vi "CAN Transceiver Test.vi"() -> ()   [LabVIEW 2024]
uses:
  Shared Modules/CAN Commands Interpreter/XNET Session Settings.ctl
  Shared Modules/CAN Commands Interpreter/CAN Frame Data.ctl
  Shared Modules/CAN Commands Interpreter/Command Values.ctl
  Type Definitions/Tester States.ctl
  Shared Modules/CAN Commands Interpreter/Target Sessions - Initialize Output Session.vi
  Shared Modules/CAN Commands Interpreter/Target Sessions - Initialize Input Session.vi
  Shared Modules/CAN Commands Interpreter/Target Sessions - Start Session.vi
  Shared Modules/CAN Commands Interpreter/Target Sessions - Stop Session.vi
  Shared Modules/CAN Commands Interpreter/Target Sessions - Clear Session.vi
  Shared Modules/CAN Commands Interpreter/CAN Commands.lvlib
panel:
  in  "Tab Control":enum32{"Sessions", "Monitor", "Errors"}(tab)
  in  "Tester Sessions":T1[](array[typedef])=[{"Interface"="CAN2", "Frame List"=["ECU_Responses\nCAN Dataframes", "HeartBit\nCAN Dataframes", "Crank_Angle\nCAN Dataframes", "Throttle\nCAN Dataframes"], "Session ID"="", "Session Name"="Tester - Read ECU Responses"}, {"Interface"="CAN2", "Frame List"=["Tester_Requests\nCAN Dataframes"], "Session ID"="", "Session Name"="Tester - Write Requests"}, {"Interface"="CAN2", "Frame List"=["HeartBit\nCAN Dataframes"], "Session ID"="", "Session Name"="Tester - Write Heartbit"}]
  out "Read ECU Data":T2[][](array[typedef]) {"ID" format="%01x"; "Payload" format="%02x"}
  in  "Command":T3={"Command"="Enable Voltage Out", "Value"=0.0}
  in  "Send Command to ECU":bool
  out "Working Mode":T4=enum."Init"
  out "Reading?":bool
  in  "STOP":bool
  out "ECU Found":bool
  out "ECU Connected":bool
  in  "Connect":bool
  in  "Disconnect":bool
  in  "Restart":bool
  out "Write Error":errorcluster
  out "Read Error":errorcluster
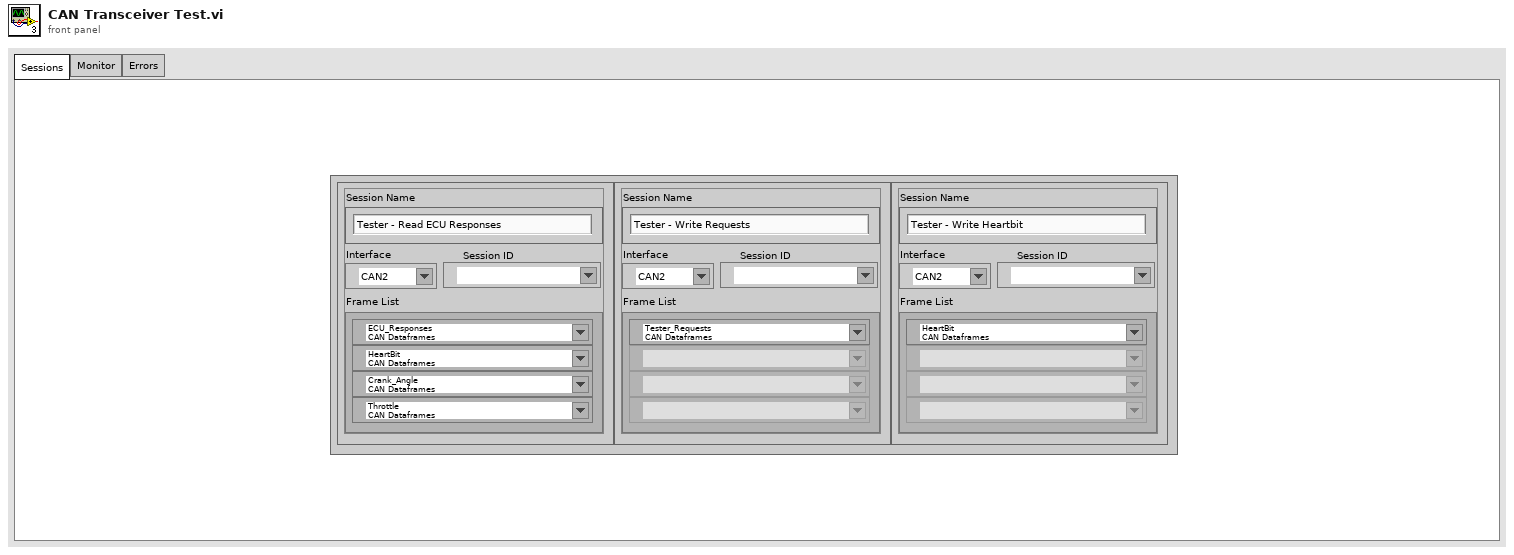
[diagram p1: front panel]
types:
  T1 = typedef "CAN Commands.lvlib/XNET Session Settings.ctl" = cluster{"Interface":refnum<k21>, "Frame List":refnum<k21>[], "Session ID":refnum<k21>, "Session Name":string}
  T2 = typedef "CAN Commands.lvlib/CAN Frame Data.ctl" = cluster{"Command":string, "XNET Frame":refnum<k21>, "Payload":u8[], "ID":u32, "Time Stamp":timestamp}
  T3 = typedef "CAN Commands.lvlib/Command Values.ctl" = cluster{"Command":string, "Value":dbl}
  T4 = typedef "Tester States.ctl" = enum16{"IDLE", "Init", "Monitoring", "Testing", "Wait for Reconnect", "Restart", "End"}
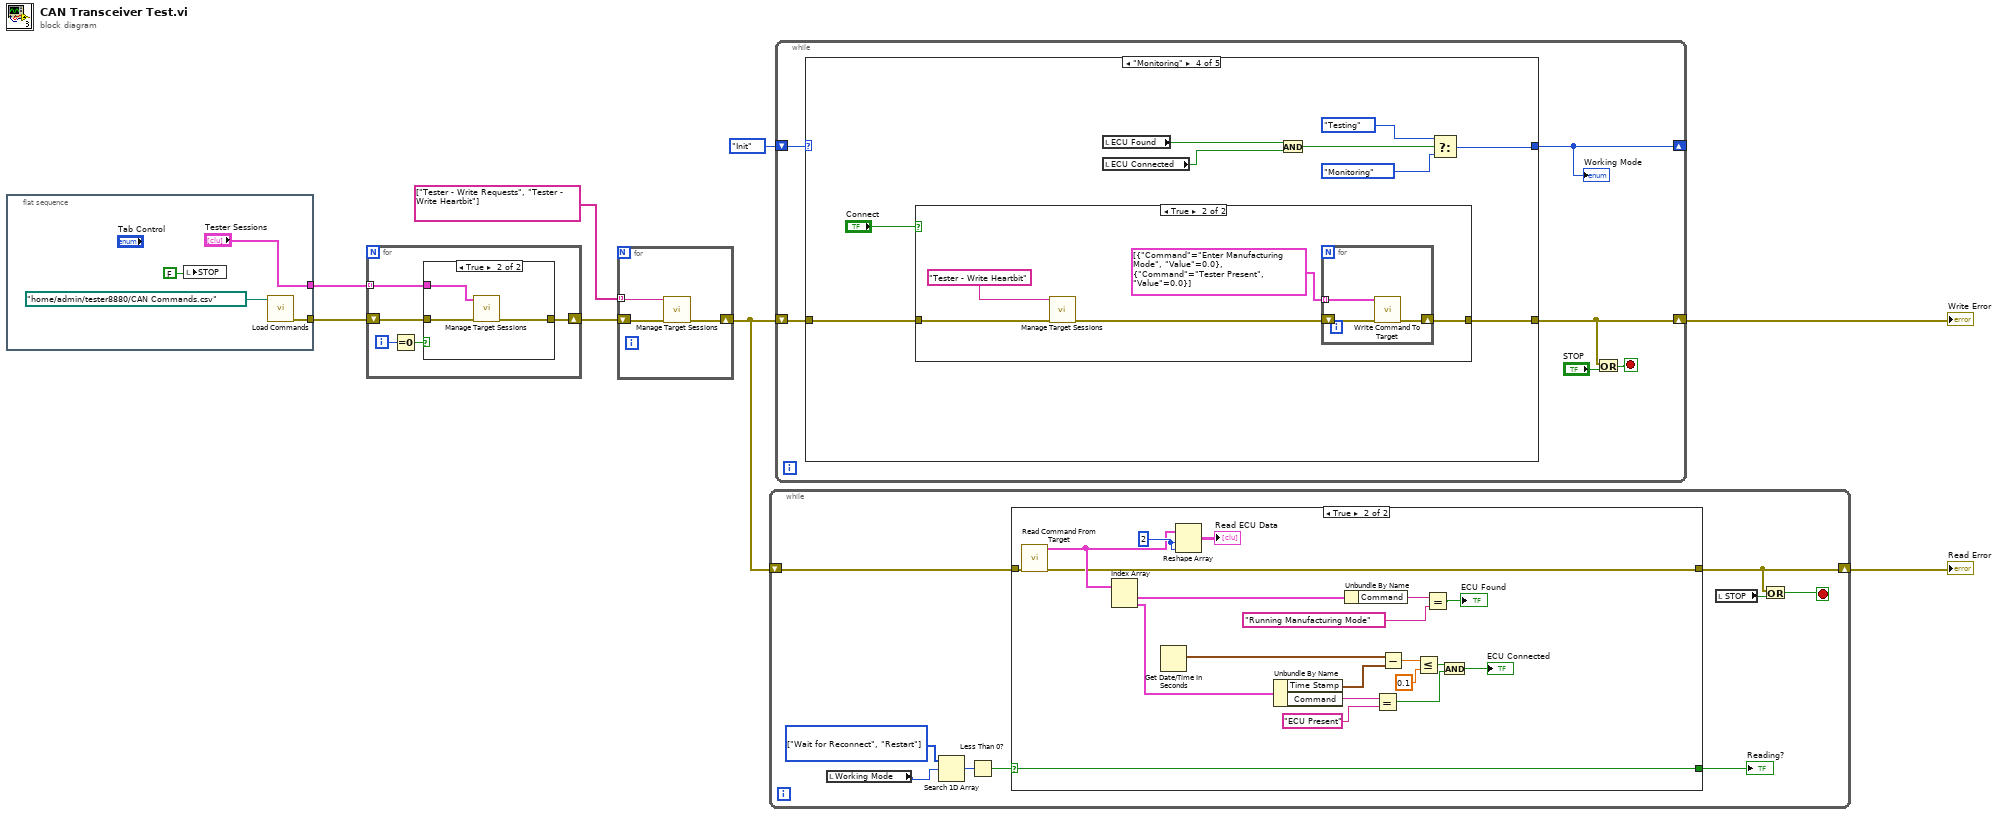
[diagram p0: block diagram]
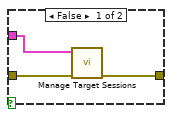
[diagram p2: hidden frame]
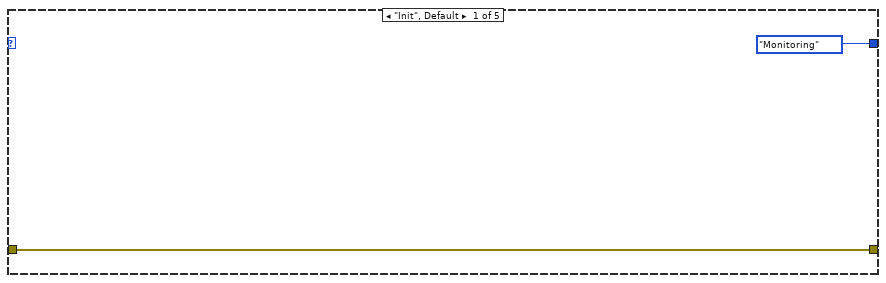
[diagram p3: hidden frame]
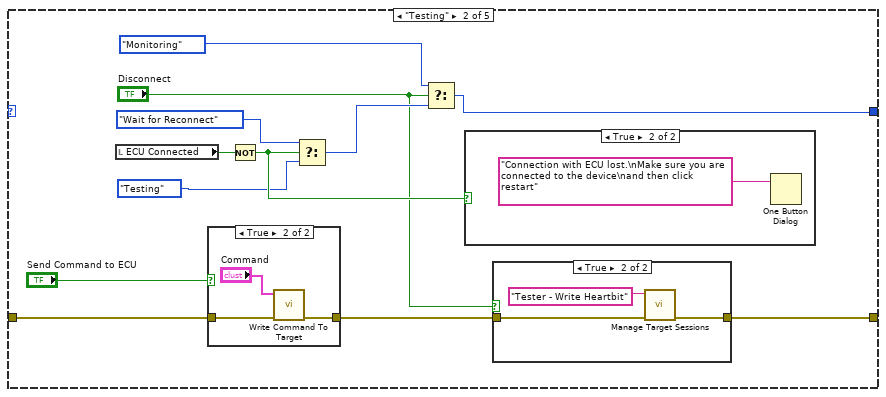
[diagram p4: hidden frame]
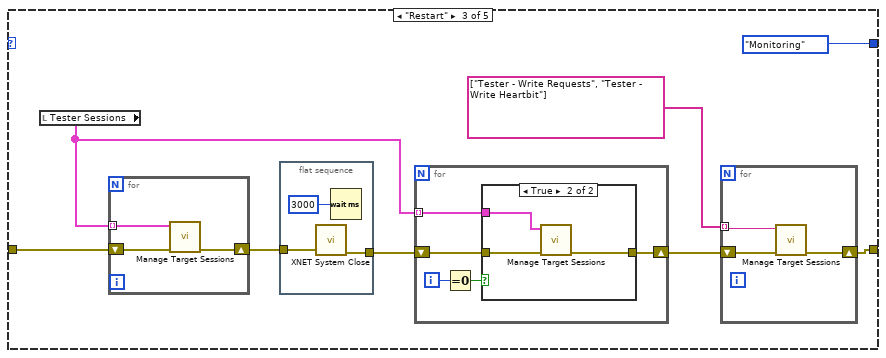
[diagram p8: hidden frame]
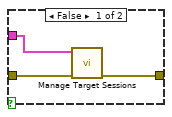
[diagram p9: hidden frame]
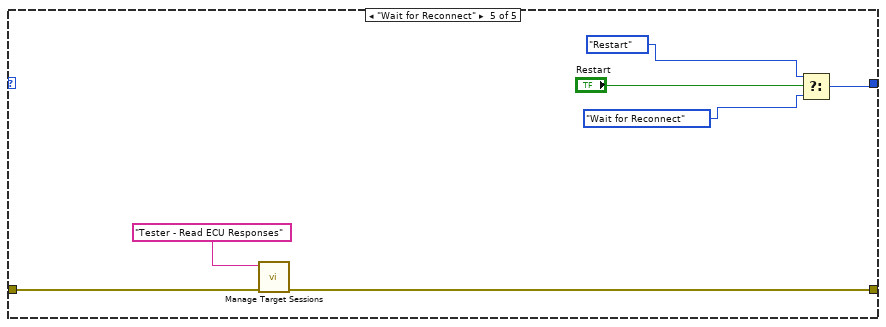
[diagram p11: hidden frame]
diagram:
  n1 = flat-sequence {
    tunnel: [w11] -> w8
    tunnel: ["Tester Sessions"] -> w4
    frame #0 {
      n2 = local write "STOP"(FALSE ("STOP")) -> ()
      n3 = call "Load Commands.vi"("Commands File (CSV)"=path "/home/admin/tester8880/CAN Commands.csv") -> ("error out"=w11:errorcluster)  [unwired: 10 in]
    }
  }
  n4 = for {
    shift-right: [w17] -> w7
    shift-left: w8 -> [w16]
    tunnel: w4 -> [w15] mode=indexing
    i -> [w13]
    n5 = Equal To 0?(x=w13) -> (x = 0?=w14:bool)
    n6 = case shown="True" w14 {
      tunnel: [w19 w23] -> w17
      tunnel: w16 -> [w20 w22]
      tunnel: w15 -> [w18 w21]
      frame False {
        n7 = call-poly "Manage Target Sessions.vi"("error in"=w20, "XNET Session Resouces"=w18) -> ("error out"=w19:errorcluster)  [unwired: 9 in]
      }
      frame True {
        n8 = call-poly "Manage Target Sessions.vi"("error in"=w22, "XNET Session Resouces"=w21) -> ("error out"=w23:errorcluster)  [unwired: 9 in]
      }
    }
  }
  n9 = for {
    shift-right: [w26] -> w1
    shift-left: w7 -> [w25]
    tunnel: string[] ["Tester - Write Requests", "Tester - Write Heartbit"] -> [w24] mode=indexing
    n10 = call-poly "Manage Target Sessions.vi"("error in"=w25, "Session Name"=w24) -> ("error out"=w26:errorcluster)  [unwired: 9 in]
  }
  n11 = while {
    shift-right: [w33] -> w5
    shift-left: w1 -> [w35]
    stop <- w32 stop-if-true
    w30 = T4[] [enum."Wait for Reconnect", enum."Restart"] items=["IDLE", "Init", "Monitoring", "Testing", "Wait for Reconnect", "Restart", "End"]
    n12 = local read "Working Mode"() -> (w29:T4)
    n13 = Search 1D Array(1D array=w30, element=w29) -> (index of element=w28:i32)  [unwired: 1 in]
    n14 = Less Than 0?(x=w28) -> (x < 0?=w27:bool)
    n15 = case shown="True" w27 {
      selector: w27 -> [_ w37]
      tunnel: w35 -> [w36 w56]
      tunnel: [w36 w38] -> w33
      tunnel: [_ w37] -> w31
      frame False {
      }
      frame True {
        w55 = 2 ("dimension size")
        n16 = call "Read Command From Target.vi"("error in"=w56) -> ("error out"=w38:errorcluster, "XNET Data"=w41:T2[])  [unwired: 7 in, 2 out]
        n17 = Index Array(array=w41) -> (element #1=w53:T2, element #2=w42:T2)  [unwired: 2 in]
        n18 = Get Date/Time In Seconds() -> (seconds since 1Jan1904=w40:timestamp)
        n19 = Reshape Array(w41, w55, w55) -> (→"Read ECU Data":T2[][])
        n20 = Unbundle By Name(w42) -> ("Time Stamp"=w43:timestamp, "Command"=w47:string)
        n21 = Unbundle By Name(w53) -> ("Command"=w52:string)
        n22 = Equal?(x=w47, y="ECU Present") -> (x = y?=w49:bool)
        n23 = Subtract(x=w40, y=w43) -> (x-y=w44:dbl)
        n24 = Less Or Equal?(x=w44, y=0.1) -> (x <= y?=w46:bool)
        n25 = Equal?(x=w52, y="Running Manufacturing Mode") -> (x = y?=→"ECU Found":bool)
        n26 = And(x=w46, y=w49) -> (x .and. y?=→"ECU Connected":bool)
      }
    }
    "Reading?" <- w31
    n27 = local read "STOP"() -> (w34:bool)
    n28 = Or(x=w33, y=w34) -> (x .or. y?=w32:bool)
  }
  "Read Error" <- w5
  n29 = while {
    shift-right: [w57] -> _
    shift-left: Tester_States."Init" -> [w62]
    shift-right: [w59] -> w2
    shift-left: w1 -> [w61]
    stop <- w58 stop-if-true
    n30 = case shown="\"Monitoring\"" w62 {
      tunnel: [Tester_States."Monitoring" w73 Tester_States."Monitoring" w118 w138] -> w57
      tunnel: [w64 w69 w87 w121 w135] -> w59
      tunnel: w61 -> [w64 w76 w88 w122 w136]
      frame "Init", Default {
      }
      frame "Testing" {
        n31 = local read "ECU Connected"() -> (w72:bool)
        n32 = case shown="True" "Send Command to ECU" {
          tunnel: w76 -> [w82 w85]
          tunnel: [w82 w84] -> w68
          frame False {
          }
          frame True {
            n33 = call "Write Command To Target.vi"("error out"=w85, "Command"="Command") -> ("error out"=w84:errorcluster)  [unwired: 9 in]
          }
        }
        n34 = Not(x=w72) -> (.not. x?=w71:bool)
        n35 = Select(t=Tester_States."Wait for Reconnect", s=w71, f=Tester_States."Testing") -> (s? t:f=w74:T4)
        n36 = Select(t=Tester_States."Monitoring", s="Disconnect", f=w74) -> (s? t:f=w73:T4)
        n37 = case shown="True" w71 {
          frame False {
          }
          frame True {
            n38 = One Button Dialog(message="Connection with ECU lost.\nMake sure you are connected to the device\nand then click restart") -> ()  [unwired: 1 in, 1 out]
          }
        }
        n39 = case shown="True" "Disconnect" {
          tunnel: [w77 w79] -> w69
          tunnel: w68 -> [w77 w78]
          frame False {
          }
          frame True {
            n40 = call-poly "Manage Target Sessions.vi"("error in"=w78, "Session Name"="Tester - Write Heartbit") -> ("error out"=w79:errorcluster)  [unwired: 9 in]
          }
        }
      }
      frame "Restart" {
        n41 = local read "Tester Sessions"() -> (w93:T1[])
        n42 = for {
          shift-right: [w113] -> w90
          shift-left: w88 -> [w112]
          tunnel: w93 -> [w111] mode=indexing
          n43 = call-poly "Manage Target Sessions.vi"("error in"=w112, "XNET Session"=w111) -> ("error out"=w113:errorcluster)  [unwired: 9 in]
        }
        n44 = flat-sequence {
          tunnel: w90 -> [w96]
          tunnel: [w95] -> w89
          frame #0 {
            n45 = call <vilib>:"XNET System Close.vi"("error in (no error)"=w96) -> ("error out"=w95:errorcluster)  [unwired: 14 in]
            n46 = Wait (ms)(milliseconds to wait=u32 3000) -> ()  [unwired: 1 out]
          }
        }
        n47 = for {
          shift-right: [w104] -> w92
          shift-left: w89 -> [w103]
          tunnel: w93 -> [w102] mode=indexing
          i -> [w100]
          n48 = Equal To 0?(x=w100) -> (x = 0?=w101:bool)
          n49 = case shown="True" w101 {
            tunnel: [w106 w110] -> w104
            tunnel: w103 -> [w107 w109]
            tunnel: w102 -> [w105 w108]
            frame False {
              n50 = call-poly "Manage Target Sessions.vi"("error in"=w107, "XNET Session Resouces"=w105) -> ("error out"=w106:errorcluster)  [unwired: 9 in]
            }
            frame True {
              n51 = call-poly "Manage Target Sessions.vi"("error in"=w109, "XNET Session Resouces"=w108) -> ("error out"=w110:errorcluster)  [unwired: 9 in]
            }
          }
        }
        n52 = for {
          shift-right: [w99] -> w87
          shift-left: w92 -> [w98]
          tunnel: string[] ["Tester - Write Requests", "Tester - Write Heartbit"] -> [w97] mode=indexing
          n53 = call-poly "Manage Target Sessions.vi"("error in"=w98, "Session Name"=w97) -> ("error out"=w99:errorcluster)  [unwired: 9 in]
        }
      }
      frame "Monitoring" {
        n54 = case shown="True" "Connect" {
          tunnel: w122 -> [w123 w126]
          tunnel: [w123 w128] -> w121
          frame False {
          }
          frame True {
            n55 = call-poly "Manage Target Sessions.vi"("error in"=w126, "Session Name"="Tester - Write Heartbit") -> ("error out"=w125:errorcluster)  [unwired: 9 in]
            n56 = for {
              shift-right: [w130] -> w128
              shift-left: w125 -> [w131]
              tunnel: T3[] [{"Command"="Enter Manufacturing Mode", "Value"=0.0}, {"Command"="Tester Present", "Value"=0.0}] -> [w129] mode=indexing
              n57 = call "Write Command To Target.vi"("error out"=w131, "Command"=w129) -> ("error out"=w130:errorcluster)  [unwired: 9 in]
            }
          }
        }
        n58 = local read "ECU Found"() -> (w120:bool)
        n59 = local read "ECU Connected"() -> (w116:bool)
        n60 = And(x=w120, y=w116) -> (x .and. y?=w117:bool)
        n61 = Select(t=Tester_States."Testing", s=w117, f=Tester_States."Monitoring") -> (s? t:f=w118:T4)
      }
      frame "Wait for Reconnect" {
        n62 = call-poly "Manage Target Sessions.vi"("error in"=w136, "Session Name"="Tester - Read ECU Responses") -> ("error out"=w135:errorcluster)  [unwired: 9 in]
        n63 = Select(t=Tester_States."Restart", s="Restart", f=Tester_States."Wait for Reconnect") -> (s? t:f=w138:T4)
      }
    }
    "Working Mode" <- w57
    n64 = Or(x=w59, y="STOP") -> (x .or. y?=w58:bool)
  }
  "Write Error" <- w2
